vi "test1.vi"   [LabVIEW 2024]
uses:
  Zero Timeout Message Handler/Zero Timeout Message Handler/Zero Timeout Message Handler.lvclass
  Zero Timeout Message Handler/Stop Msg/Stop Msg.lvclass
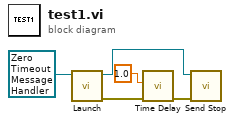
[diagram p0: block diagram]
diagram:
  n1 = call "Launch.vi"("Zero Timeout Message Handler in"=refnum<class "Zero Timeout Message Handler.lvclass"> refnum) -> ("error out"=w4:errorcluster, "Message Queue"=w1:refnum<queue>)  [unwired: 9 in]
  n2 = call "Time Delay"("error in (no error)"=w4, "Delay Time (s)"=1.0) -> ("error out"=w3:errorcluster)  [unwired: 9 in]
  n3 = call "Send Stop.vi"("error in (no error)"=w3, "Message Queue"=w1) -> ()  [unwired: 9 in, 1 out]
